vi "GmailLV89.vi"(7 "string":string, 8 "Body":string) -> ()   [LabVIEW 2013]
panel:
  in  "Attachment - Optional":path
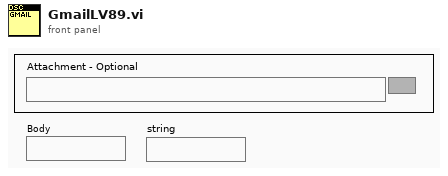
[diagram p1: front panel]
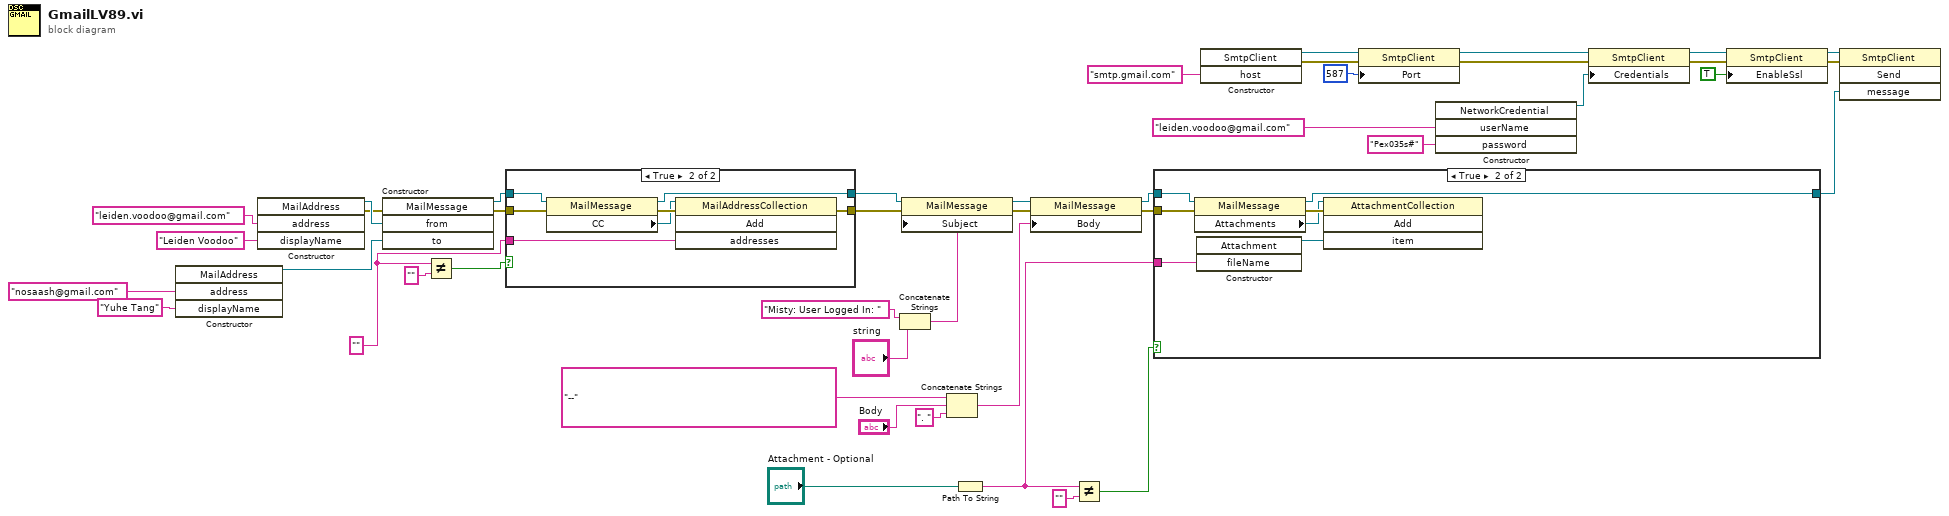
[diagram p0: block diagram]
diagram:
  w17 = "" ("CC - Optional")
  n1 = constructor class="MailAddress"("address"="nosaash@gmail.com" ("Recipient's Email Address"), "displayName"="Yuhe Tang" ("Recipient's Name")) -> (reference out=w44:refnum<k24>)  [unwired: 3 in, 4 out]
  n2 = constructor class="MailAddress"("address"="leiden.voodoo@gmail.com" ("Sender's Email Address (eg: LabVIEW@gmail.com)"), "displayName"="Leiden Voodoo" ("Sender's Name")) -> (reference out=w43:refnum<k24>, error out=w9:errorcluster)  [unwired: 3 in, 3 out]
  n3 = constructor class="MailMessage"(error in=w9, "from"=w43, "to"=w44) -> (reference out=w16:refnum<k24>, error out=w15:errorcluster)  [unwired: 2 in, 3 out]
  n4 = Not Equal?(x=w17, y="") -> (x != y?=w18:bool)
  n5 = case shown="True" w18 {
    tunnel: w17 -> [_ w51]
    tunnel: w16 -> [w46 w50]
    tunnel: w15 -> [w45 w49]
    tunnel: [w46 w48] -> w14
    tunnel: [w45 w47] -> w13
    frame False {
    }
    frame True {
      n6 = property class="MailMessage"(reference=w50, error in=w49) -> (reference out=w48:refnum<k24>, error out=w53:errorcluster, "CC"=w52:refnum<k24>)
      n7 = invoke class="MailAddressCollection" method="Add"(reference=w52, error in=w53, "addresses"=w51) -> (error out=w47:errorcluster)  [unwired: 1 in, 3 out]
    }
  }
  n8 = Concatenate Strings("Misty: User Logged In: " ("Subject"), "string") -> (w2:string)
  n9 = property class="MailMessage"(reference=w14, error in=w13, "Subject"=w2) -> (reference out=w36:refnum<k24>, error out=w42:errorcluster)
  n10 = Concatenate Strings("--" ("string"), "Body", ". " ("string")) -> (w6:string)
  n11 = Path To String(path="Attachment - Optional") -> (string=w20:string)
  n12 = property class="MailMessage"(reference=w36, error in=w42, "Body"=w6) -> (reference out=w24:refnum<k24>, error out=w8:errorcluster)
  n13 = Not Equal?(x=w20, y="") -> (x != y?=w21:bool)
  n14 = case shown="True" w21 {
    tunnel: w24 -> [w54 w58]
    tunnel: [w54 w57] -> w12
    tunnel: w20 -> [_ w56]
    tunnel: w8 -> [_ w55]
    frame False {
    }
    frame True {
      n15 = property class="MailMessage"(reference=w58, error in=w55) -> (reference out=w57:refnum<k24>, error out=w61:errorcluster, "Attachments"=w59:refnum<k24>)
      n16 = constructor class="Attachment"("fileName"=w56) -> (reference out=w60:refnum<k24>)  [unwired: 3 in, 3 out]
      n17 = invoke class="AttachmentCollection" method="Add"(reference=w59, error in=w61, "item"=w60) -> ()  [unwired: 1 in, 4 out]
    }
  }
  n18 = constructor class="SmtpClient"("host"="smtp.gmail.com" ("Outgoing Mail Server (SMTP)")) -> (reference out=w30:refnum<k24>, error out=w27:errorcluster)  [unwired: 3 in, 2 out]
  n19 = property class="SmtpClient"(reference=w30, error in=w27, "Port"=587) -> (reference out=w29:refnum<k24>, error out=w26:errorcluster)
  n20 = constructor class="NetworkCredential"("userName"="leiden.voodoo@gmail.com" ("GMAIL Account User ID"), "password"="Pex035s#" ("GMAIL Account Password")) -> (reference out=w31:refnum<k24>)  [unwired: 3 in, 4 out]
  n21 = property class="SmtpClient"(reference=w29, error in=w26, "Credentials"=w31) -> (reference out=w28:refnum<k24>, error out=w25:errorcluster)
  n22 = property class="SmtpClient"(reference=w28, error in=w25, "EnableSsl"=TRUE ("Enable SSL")) -> (reference out=w10:refnum<k24>, error out=w11:errorcluster)
  n23 = invoke class="SmtpClient" method="Send"(reference=w10, error in=w11, "message"=w12) -> ()  [unwired: 1 in, 4 out]
